vi "sub_read_string_from_JSON_file.vi"(8 "error in (no error)":errorcluster, 11 "appended path":path) -> (0 "error out":errorcluster, 3 "Value":string)   [LabVIEW 2013, in "daqio minimal.lvlib"]
uses:
  daqio minimal.lvlib
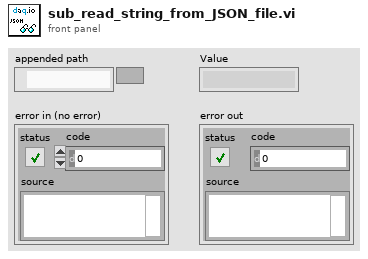
[diagram p1: front panel]
types:
  T1 = enum16{"open", "replace", "create", "open or create", "replace or create", "replace or create with confirmation"}
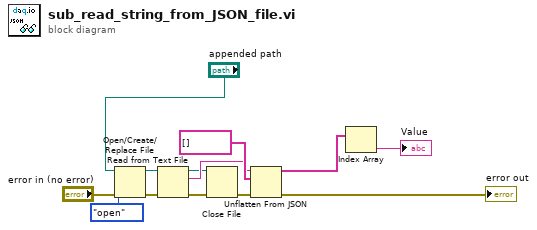
[diagram p0: block diagram]
diagram:
  n1 = Open/Create/Replace File(file path (use dialog)="appended path", error in="error in (no error)", operation (0:open)=T1."open") -> (refnum out=w7:refnum<file>, error out=w4:errorcluster)  [unwired: 3 in, 1 out]
  n2 = Read from Text File(file (use dialog)=w7, error in=w4) -> (refnum out=w6:refnum<file>, text=w9:string, error out=w5:errorcluster)  [unwired: 2 in, 1 out]
  n3 = Close File(refnum=w6, error in=w5) -> (error out=w8:errorcluster)  [unwired: 1 out]
  n4 = Unflatten From JSON(JSON string=w9, type and defaults=string[] [], error in (no error)=w8) -> (value=w12:string[], error out=→"error out":errorcluster)  [unwired: 4 in]
  n5 = Index Array(array=w12) -> (element=→"Value":string)  [unwired: 1 in]
